vi "Control Mode Read Single.vi"(8 "error in":errorcluster, 9 "Channel Index":i32, 11 "Chiller In":refnum<class "Chiller.lvclass">) -> (0 "error out":errorcluster, 1 "Changed or First Call?":bool, 2 "Control Mode CTL":u16, 3 "Chiller out":refnum<class "Chiller.lvclass">)   [LabVIEW 2023, in "Chiller.lvclass"]
uses:
  Chiller.lvclass
  Chiller.lvclass/Chiller.ctl
  Low Level Capabilities/Control Mode/Control Mode.lvclass
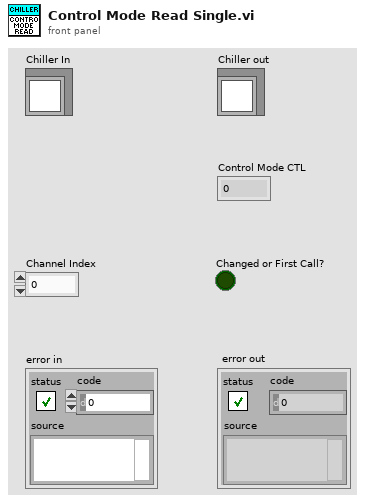
[diagram p1: front panel]
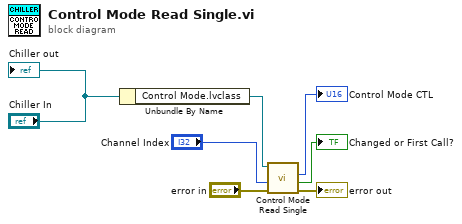
[diagram p0: block diagram]
diagram:
  n1 = Unbundle By Name("Chiller In") -> ("Control Mode.lvclass"=w2:refnum<class "Control Mode.lvclass">)
  n2 = call-dynamic "Control Mode Read Single.vi"("error in"="error in", "Channel Index"="Channel Index", "Control Mode in"=w2) -> ("error out"=→"error out":errorcluster, "Changed or First Call?"=→"Changed or First Call?":bool, "Control Mode CTL"=→"Control Mode CTL":u16)  [unwired: 5 in, 1 out]
  "Chiller out" <- "Chiller In"
